vi "Play Path.vi"(6 "Reset Gyro":bool=TRUE, 11 "Path Name":string="BarrelFastCarpet") -> ()   [LabVIEW 2019]
uses:
  Implementation/Drive Base Operations.ctl
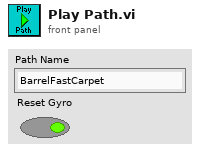
[diagram p1: front panel]
types:
  T1 = typedef "Drive Base Operations.ctl" = enum16{"Reserve", "Read Current", "Immediate", "Limelight", "Manual Adjustment", "Play Path"}
  T2 = cluster{"Segment Name":string, "Type":enum16{"Accel Straight", "Const Straight", "Blend", "Circle"}, "Traj Pos Points":cluster{"x":dbl, "y":dbl, "th":dbl}[], "Traj Vel Points":cluster{"V":dbl, "th":dbl}[], "Accel Index":i32, "Decel Index":i32}[]
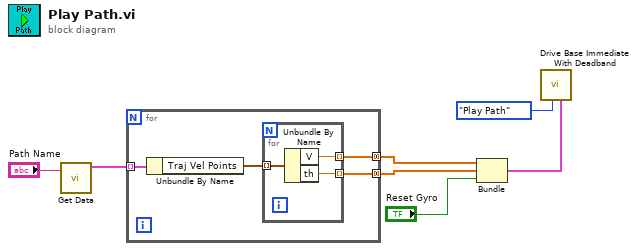
[diagram p0: block diagram]
diagram:
  n1 = call "Get Data.vi"("Path Name"="Path Name") -> ("Trajectory Data"=w6:T2)  [unwired: 8 in, 2 out]
  n2 = for {
    tunnel: w6 -> [w11] mode=indexing
    tunnel: [w9] -> w4 mode=concatenating
    tunnel: [w8] -> w3 mode=concatenating
    n3 = Unbundle By Name(w11) -> ("Traj Vel Points"=w10:cluster{"V":dbl, "th":dbl}[])
    n4 = for {
      tunnel: w10 -> [w14] mode=indexing
      tunnel: [w13] -> w9 mode=indexing
      tunnel: [w12] -> w8 mode=indexing
      n5 = Unbundle By Name(w14) -> ("V"=w13:dbl, "th"=w12:dbl)
    }
  }
  n6 = Bundle(w4, w3, "Reset Gyro"="Reset Gyro") -> (w2:cluster{dbl[], dbl[], "Reset Gyro":bool})  [unwired: 1 in]
  n7 = call "Drive Base Immediate With Deadband.vi"("Path Planner Data"=w2, "Operation"=Drive_Base_Operations."Play Path") -> ()  [unwired: 9 in, 1 out]
